vi "chart set table grid.vi"(6 "legend_keys":u8, 7 "outline":u8, 8 "error in (no error)":errorcluster, 9 "vertical":u8, 10 "horizontal":u8, 11 "chart":u32) -> (0 "error out":errorcluster)   [LabVIEW 2015, in "xlsxwriter.lvlib"]
doc: "void chart_set_table_grid(lxw_chart chart, uint8_t horizontal, uint8_t vertical, uint8_t outline, uint8_t legend_keys);"
uses:
  xlsxwriter.lvlib
  xlsxwriter.dll
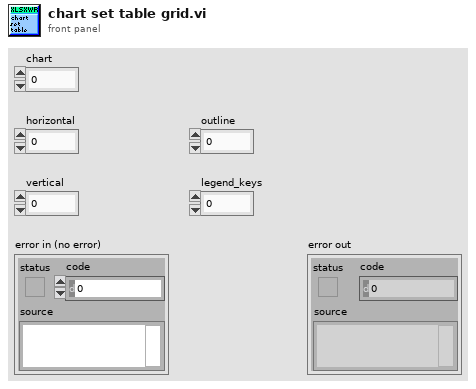
[diagram p1: front panel]
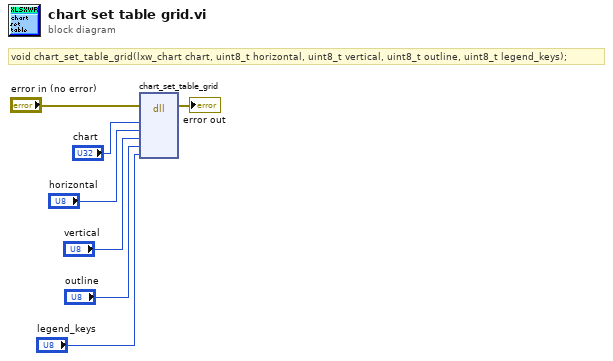
[diagram p0: block diagram]
diagram:
  # "void chart_set_table_grid(lxw_chart chart, uint8_t horizontal, uint8_t vertical, uint8_t outline, uint8_t legend_keys);"
  n1 = dll-call lib="C:/Users/WDAGUtilityAccount/Desktop/lv_vis_added_cell/xlsxwriter.*" fn="chart_set_table_grid"(error in="error in (no error)", "chart"="chart", "horizontal"="horizontal", "vertical"="vertical", "outline"="outline", "legend_keys"="legend_keys") -> (error out=→"error out":errorcluster)  [unwired: 8 in, 1 out]
